vi "c ctre phoenixpro get signal simplified.vi"(0 "network":string, 1 "device_hashes":u32[](array[numeric])=array[4097 elements], 5 "bWaitForUpdate":i32, 7 "timeoutSeconds":dbl, 9 "num_signals":u32, 11 "error in (no error)":errorcluster, 12 "spns":u32[](array[numeric])=array[4097 elements]) -> (3 "function return":i32, 4 "values":dbl[](array[numeric]), 6 "hwTimestampSeconds":dbl[](array[numeric]), 8 "swTimestampSeconds":dbl[](array[numeric]), 10 "ecuTimestampSeconds":dbl[](array[numeric]), 15 "error out":errorcluster)   [LabVIEW 2020, in "CTRE_PhoenixTools.lvlib"]
doc: "CTREXPORT int c_ctre_phoenixpro_get_signal_simplified(\n \n const char *network,\n int bWaitForUpdate,\n double timeoutSeconds,\n \n uint32_t num_signals,\n const uint32_t *device_hashes, const uint32_t *spns, \n double *values, double *hwTimestampSeconds, double *swTimestampSeconds, double *ecuTimestampSeconds );"
uses:
  <userlib>/CTRE_PhoenixTools/CTRE_PhoenixTools.lvlib
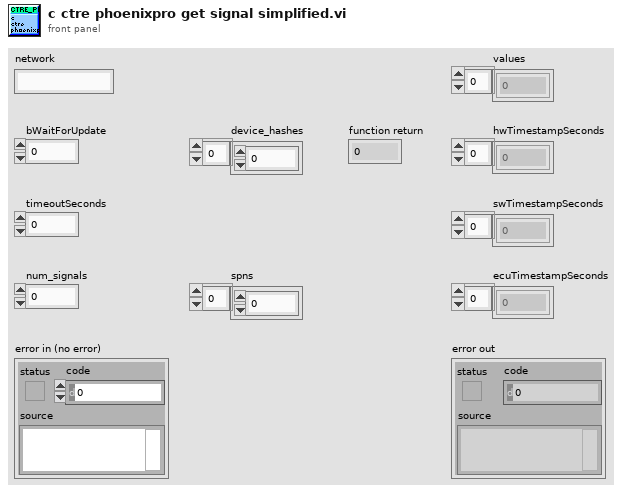
[diagram p1: front panel]
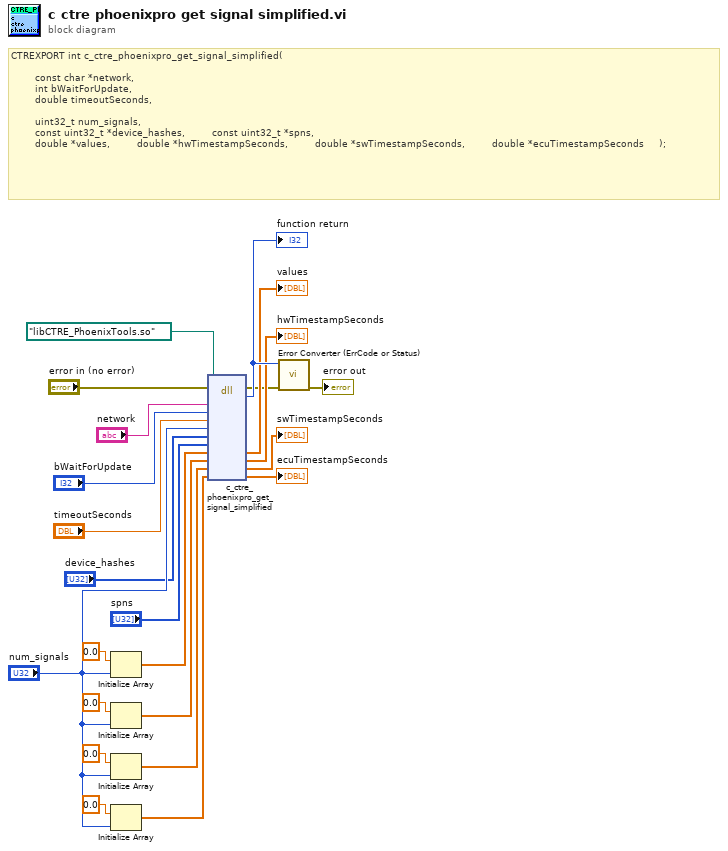
[diagram p0: block diagram]
diagram:
  # "CTREXPORT int c_ctre_phoenixpro_get_signal_simplified(\n        \n        const char *network,\n        int bWaitForUpdate,\n        double timeoutSeconds,\n        \n        uint32_t num_signals,\n        const uint32_t *device_hashes,         const uint32_t *spns,         \n        double *values,         double *hwTimestampSeconds,         double *swTimestampSeconds,         double *ecuTimestampSeconds     );"
  n1 = Initialize Array(0.0 ("element"), "num_signals") -> (w16:dbl[])
  n2 = Initialize Array(0.0 ("element"), "num_signals") -> (w13:dbl[])
  n3 = Initialize Array(0.0 ("element"), "num_signals") -> (w10:dbl[])
  n4 = Initialize Array(0.0 ("element"), "num_signals") -> (w7:dbl[])
  n5 = dll-call lib="?" fn="c_ctre_phoenixpro_get_signal_simplified"(path in=path "libCTRE_PhoenixTools.so", error in="error in (no error)", "network"="network", "bWaitForUpdate"="bWaitForUpdate", "timeoutSeconds"="timeoutSeconds", "num_signals"="num_signals", "device_hashes"="device_hashes", "spns"="spns", "values"=w16, "hwTimestampSeconds"=w13, "swTimestampSeconds"=w10, "ecuTimestampSeconds"=w7) -> (error out=w3:errorcluster, "return type"=w23:i32, "values"=→"values":dbl[], "hwTimestampSeconds"=→"hwTimestampSeconds":dbl[], "swTimestampSeconds"=→"swTimestampSeconds":dbl[], "ecuTimestampSeconds"=→"ecuTimestampSeconds":dbl[])  [unwired: 7 in, 1 out]
  "function return" <- w23
  n6 = call <userlib>:"Error Converter (ErrCode or Status).vi"("error in (no error)"=w3, "error code"=w23) -> ("error out"=→"error out":errorcluster)  [unwired: 9 in]
